vi "Firmware Wizard Check INI.vi"(8 "Error In":errorcluster) -> (0 "Error Out":errorcluster)   [LabVIEW 2020, in "LMH-LINX.lvlib"]
uses:
  LMH-LINX.lvlib
  <vilib>/Utility/config.llb/Write Key (Path).vi
  Toolbox/LMH-Toolbox.lvlib
  <vilib>/Utility/config.llb/NI_LVConfig.lvlib
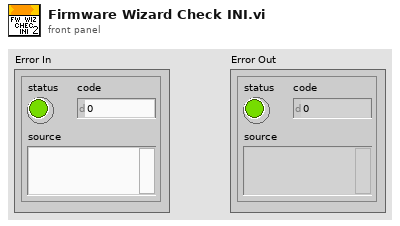
[diagram p1: front panel]
types:
  T1 = typedef "NI_LVConfig.lvlib/Config Data RefNum.ctl" = refnum<k1>
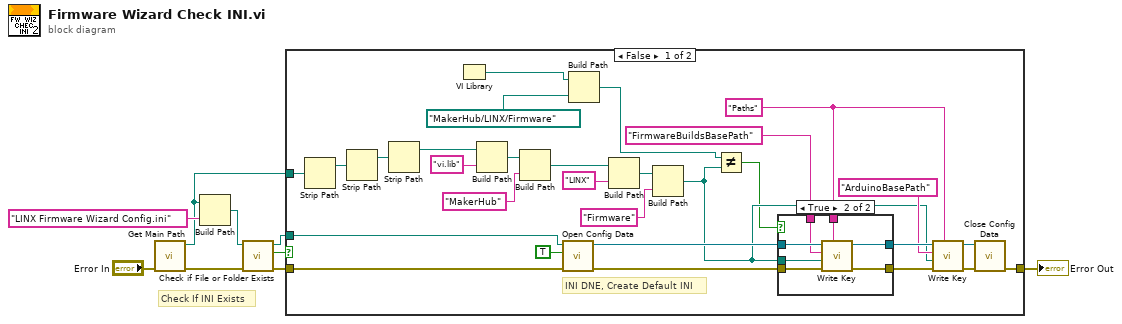
[diagram p0: block diagram]
diagram:
  # "Check If INI Exists"
  n1 = call "Get Main Path.vi"("Error In"="Error In") -> ("Error Out"=w9:errorcluster, "Main Dir"=w2:path)  [unwired: 8 in, 1 out]
  n2 = Build Path(base path=w2, name or relative path="LINX Firmware Wizard Config.ini") -> (appended path=w6:path)
  n3 = call <vilib>:"Check if File or Folder Exists.vi"("error in (no error)"=w9, "path"=w6) -> ("error out"=w5:errorcluster, "file or folder exists?"=w4:bool, "dup path"=w1:path)  [unwired: 7 in]
  n4 = case shown="False" w4 {
    tunnel: w5 -> [w34 w48]
    tunnel: [w31 w48] -> w3
    tunnel: w2 -> [w33 _]
    tunnel: w1 -> [w30 _]
    frame False {
      w18 = "Paths" ("section")
      # "INI DNE, Create Default INI"
      n5 = Strip Path(path=w33) -> (stripped path=w29:path)  [unwired: 1 out]
      n6 = Strip Path(path=w29) -> (stripped path=w28:path)  [unwired: 1 out]
      n7 = Strip Path(path=w28) -> (stripped path=w27:path)  [unwired: 1 out]
      n8 = VI Library() -> (path=w13:path)
      n9 = Build Path(base path=w27, name or relative path="vi.lib") -> (appended path=w25:path)
      n10 = Build Path(base path=w25, name or relative path="MakerHub") -> (appended path=w23:path)
      n11 = call <vilib>:"Open Config Data.vi"("error in (no error)"=w34, "create file if necessary (T)"=TRUE, "configuration file path"=w30) -> ("error out"=w38:errorcluster, "refnum"=w37:T1)  [unwired: 6 in, 1 out]
      n12 = Build Path(base path=w13, name or relative path=path "MakerHub/LINX/Firmware") -> (appended path=w11:path)
      n13 = Build Path(base path=w23, name or relative path="LINX") -> (appended path=w21:path)
      n14 = Build Path(base path=w21, name or relative path="Firmware") -> (appended path=w12:path)
      n15 = Not Equal?(x=w11, y=w12) -> (x != y?=w10:bool)
      n16 = case shown="True" w10 {
        tunnel: w38 -> [w39 w47]
        tunnel: w37 -> [w40 w46]
        tunnel: "FirmwareBuildsBasePath" ("key") -> [_ w45]
        tunnel: [w40 w44] -> w20
        tunnel: [w39 w43] -> w19
        tunnel: w18 -> [_ w42]
        tunnel: w12 -> [_ w41]
        frame False {
        }
        frame True {
          n17 = call-poly <vilib>:"Write Key.vi"("section"=w42, "error in (no error)"=w47, "value"=w41, "key"=w45, "refnum"=w46) -> ("error out"=w43:errorcluster, "refnum out"=w44:T1)  [unwired: 4 in, 1 out]
        }
      }
      n18 = call-poly <vilib>:"Write Key.vi"("section"=w18, "error in (no error)"=w19, "value"=w12, "key"="ArduinoBasePath", "refnum"=w20) -> ("error out"=w15:errorcluster, "refnum out"=w16:T1)  [unwired: 4 in, 1 out]
      n19 = call <vilib>:"Close Config Data.vi"("error in (no error)"=w15, "refnum"=w16) -> ("error out"=w31:errorcluster)  [unwired: 8 in, 1 out]
    }
    frame True {
      # "INI Exists, Nothing To Do"
    }
  }
  "Error Out" <- w3
